vi "PUMPCONFIG07_2.vi"(0 "?":bool, 1 "Radio Buttons":enum32{"Reglo Digital", "Reglo Analog", "PAM"}(radio), 2 "Bypass (g/min)":dbl, 5 "Target (g) in":dbl, 7 "Amount (g)":dbl, 9 "Time (min) in":dbl, 11 "Flow rate in":dbl, 12 "OK Button":bool, 13 "Port":i32=15) -> (3 "Time to target 2":dbl format="%<%H:%M:%S>t", 4 "Time to target":dbl format="%<%H:%M:%S>t", 6 "mA":dbl format="%#_2g", 8 "signal":dbl, 10 "Speed":dbl, 14 "RPM":dbl format="%#_2g", 15 "Array":bool[](array[boolean]))   [LabVIEW 2015]
uses:
  x64/Debug/BERTTA.dll
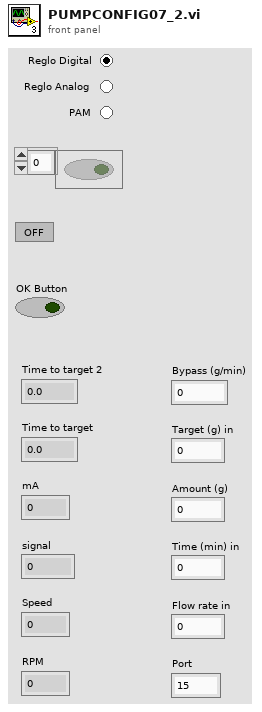
[diagram p1: front panel]
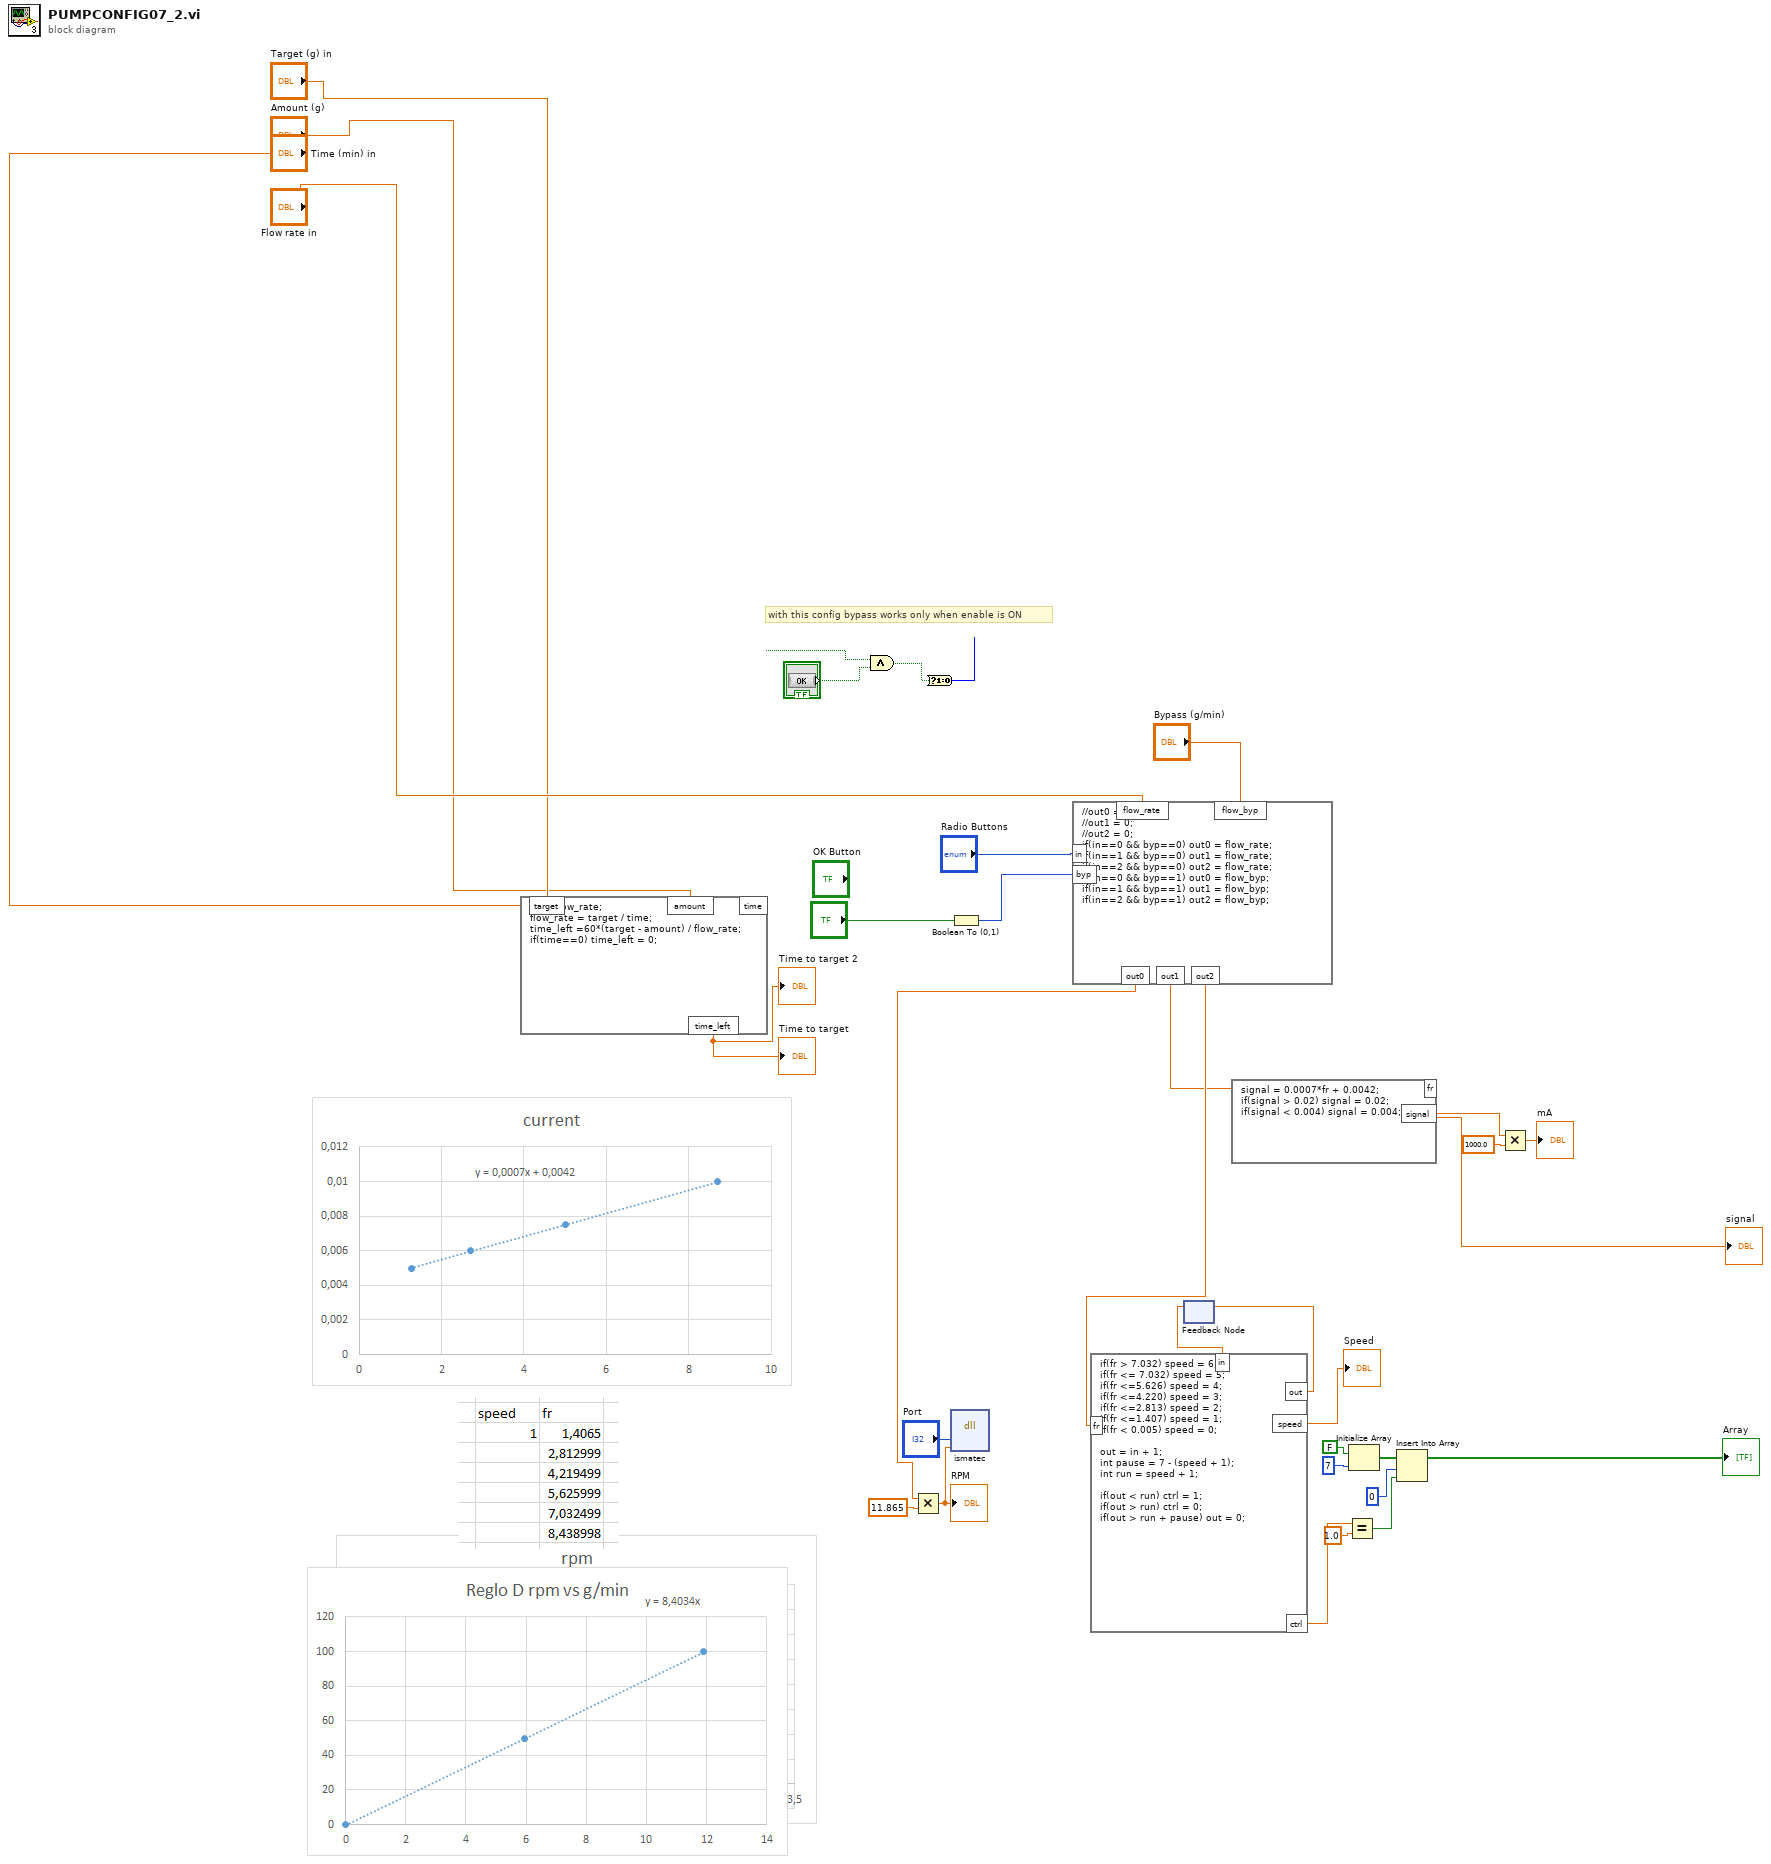
[diagram p0: block diagram]
diagram:
  # "with this config bypass works only when enable is ON"
  n1 = formula code="float flow_rate;\nflow_rate = target / time;\ntime_left =60*(target - amount) / flow_rate;\nif(time==0) time_left = 0;"("target"="Target (g) in", "amount"="Amount (g)", "time"="Time (min) in") -> ("time_left"=→"Time to target" →"Time to target 2":dbl)
  n2 = Boolean To (0,1)(Boolean="?") -> (0, 1=w20:i16)
  n3 = formula code="//out0 = 0;\n//out1 = 0;\n//out2 = 0;\nif(in==0 && byp==0) out0 = flow_rate;\nif(in==1 && byp==0) out1 = flow_rate;\nif(in==2 && byp==0) out2 = flow_rate;\nif(in==0 && byp==1) out0 = flow_byp;\nif(in==1 && byp==1) out1 = flow_byp;\nif(in==2 && byp==1) out2 = flow_byp;"("in"="Radio Buttons", "flow_rate"="Flow rate in", "flow_byp"="Bypass (g/min)", "byp"=w20) -> ("out0"=w23:dbl, "out1"=w21:dbl, "out2"=w22:dbl)
  n4 = Multiply(x=w23, y=11.865) -> (x*y=w16:dbl)
  "RPM" <- w16
  n5 = dll-call lib="C:/Users/shresplab/OneDrive - Kemira Oyj/Documents/Visual Studio 2017/Projects/Bertta/BERTTA/x64/Debug/BERTTA.dll" fn="ismatec"("port"="Port", "speed"=w16) -> ()  [unwired: 6 in, 2 out]
  n6 = feedback #1() -> (w8:dbl)  [unwired: 1 in]
  n7 = formula code="if(fr > 7.032) speed = 6;\nif(fr <= 7.032) speed = 5;\nif(fr <=5.626) speed = 4;\nif(fr <=4.220) speed = 3;\nif(fr <=2.813) speed = 2;\nif(fr <=1.407) speed = 1;\nif(fr < 0.005) speed = 0;\n\nout = in + 1;\nint pause = 7 - (speed + 1);\nint run = speed + 1;\n\nif(out < run) ctrl = 1;\nif(out > run) ctrl = 0;\nif(out > run + pause) out = 0;"("in"=w8, "fr"=w22) -> ("out"=w7:dbl, "ctrl"=w9:dbl, "speed"=→"Speed":dbl)
  n8 = feedback-in #1(w7) -> ()
  n9 = formula code="signal = 0.0007*fr + 0.0042;\nif(signal > 0.02) signal = 0.02;\nif(signal < 0.004) signal = 0.004;"("fr"=w21) -> ("signal"=w13:dbl)
  "signal" <- w13
  n10 = Equal?(x=w9, y=1.0) -> (x = y?=w11:bool)
  n11 = Initialize Array(FALSE, 7 ("dimension size")) -> (w4:bool[])
  n12 = Insert Into Array(array=w4, index=0, new element=w11) -> (→"Array":bool[])
  n13 = Multiply(x=w13, y=1000.0) -> (x*y=→"mA":dbl)
